vi "Read Timeout (ms).vi"(8 "error in (no error)":errorcluster, 11 "WebSocket Connection in":refnum<class "WebSocket Connection.lvclass">) -> (0 "error out":errorcluster, 2 "Timeout (ms)":i32=5000, 3 "WebSocket Connection out":refnum<class "WebSocket Connection.lvclass">)   [LabVIEW 2016, in "WebSocket Actors.lvlib" / "WebSocket Connection.lvclass"]
uses:
  WebSocket Connection.lvclass
  WebSocket Connection.lvclass/WebSocket Connection.ctl
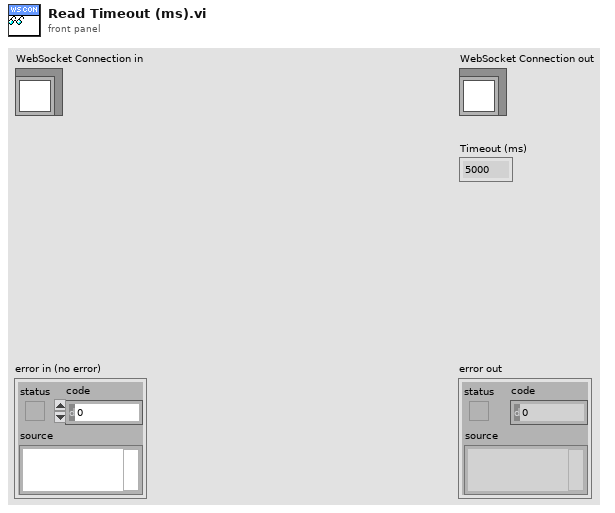
[diagram p1: front panel]
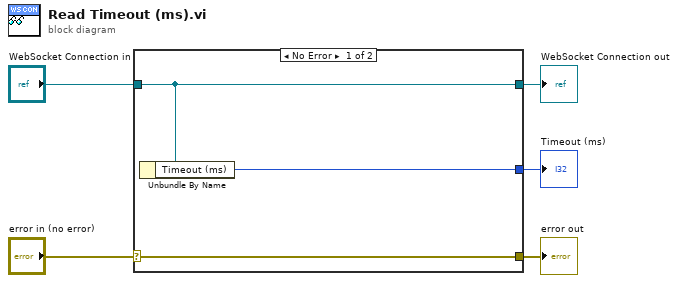
[diagram p0: block diagram]
diagram:
  n1 = case shown="No Error" "error in (no error)" {
    selector: "error in (no error)" -> [w8 w9]
    tunnel: [w8 w9] -> w4
    tunnel: [w7 w10] -> w2
    tunnel: "WebSocket Connection in" -> [w7 w10]
    tunnel: [w6 _] -> w1
    frame No Error {
      n2 = Unbundle By Name(w7) -> ("Timeout (ms)"=w6:i32)
    }
    frame Error {
    }
  }
  "error out" <- w4
  "WebSocket Connection out" <- w2
  "Timeout (ms)" <- w1
